vi "OpenNRun.vi"(1 "VI name":string, 2 "ViDirPath":path) -> (0 "Execution:State":T1(ring))   [LabVIEW 2015]
panel:
  out "complete path":path
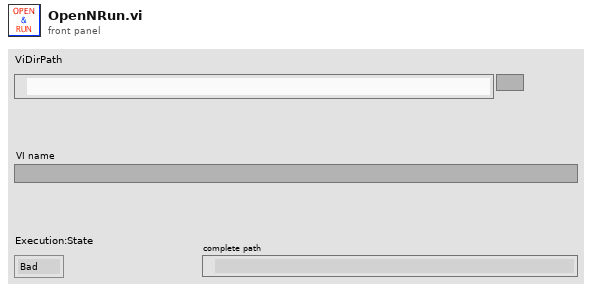
[diagram p1: front panel]
types:
  T1 = enum32{"Bad", "Idle", "Run top level", "Running"}
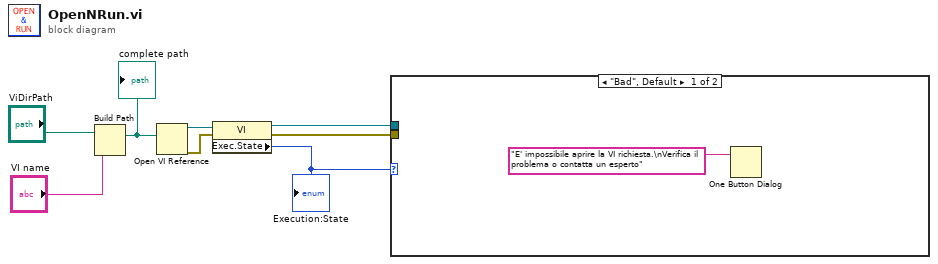
[diagram p0: block diagram]
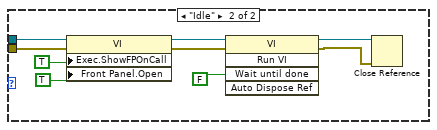
[diagram p2: hidden frame]
diagram:
  n1 = Build Path(base path="ViDirPath", name or relative path="VI name") -> (appended path=w5:path)
  "complete path" <- w5
  n2 = Open VI Reference(vi path=w5) -> (vi reference=w4:refnum<vi>, error out=w3:errorcluster)  [unwired: 5 in]
  n3 = property class="VI"(reference=w4, error in=w3) -> (reference out=w2:refnum<vi>, error out=w1:errorcluster, "Exec.State"=w6:T1)
  "Execution:State" <- w6
  n4 = case shown="\"Bad\", Default" w6 {
    tunnel: w2 -> [_ w14]
    tunnel: w1 -> [_ w13]
    frame "Bad", Default {
      n5 = One Button Dialog(message="E' impossibile aprire la VI richiesta.\nVerifica il problema o contatta un esperto") -> ()  [unwired: 1 in, 1 out]
    }
    frame "Idle" {
      n6 = property class="VI"(reference=w14, error in=w13, "Exec.ShowFPOnCall"=TRUE ("Execution:Show Front Panel On Load"), "Front Panel.Open"=TRUE ("Front Panel Window:Open")) -> (reference out=w15:refnum<vi>, error out=w12:errorcluster)
      n7 = invoke class="VI" method="Run VI"(reference=w15, error in=w12, "Wait until done"=FALSE ("Wait Until Done")) -> (reference out=w11:refnum<vi>, error out=w10:errorcluster)  [unwired: 2 in, 3 out]
      n8 = Close Reference(reference=w11, error in (no error)=w10) -> ()  [unwired: 1 out]
    }
  }
